vi "Feet to Encoder Value.vi"(1 "Feet":dbl) -> (0 "Encoder Value":dbl)   [LabVIEW 2017]
doc: "Takes a numeric input, divides it by 1.57 and multiplies the quotient by 4096(encoder rotation)."
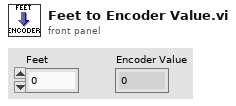
[diagram p1: front panel]
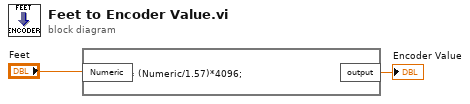
[diagram p0: block diagram]
diagram:
  n1 = formula code="output = (Numeric/1.57)*4096;"("Numeric"="Feet") -> ("output"=→"Encoder Value":dbl)
